vi "SLM_Calibrator.vi"() -> ()   [LabVIEW 2011]
uses:
  <vilib>/userDefined/High Color/IMAQdx.ctl
  <vilib>/vision/driver/NI_Vision_Acquisition_Software.lvlib
panel:
  in  "Xoffset2":dbl=4.136690647482014
  in  "Yoffset2":dbl=4.136690647482014
  in  "Yoffset1":dbl=6.374501992031872 caption="Fine:"
  in  "Xoffset1":dbl=6.374501992031872 caption="Fine:"
  in  "Direct to MatLab":bool
  out "ph_2_135":bool
  out "ph_2_45":bool
  out "ph_1_135":bool
  out "ph_1_45":bool
  out "I_2":bool
  out "I_1":bool
  out "0_255":dbl[](array[numeric])
  out "SupportFiles path":path
  out "I2":dbl[](array[numeric])
  out "ph2 135":dbl[](array[numeric])
  out "ph2 45":dbl[](array[numeric])
  out "I1":dbl[](array[numeric])
  out "ph1 135":dbl[](array[numeric])
  out "ph1_45":dbl[](array[numeric])
  in  "Ready?\nCalibrate!":bool caption="Stop (F)"
  in  "Active2":bool=TRUE caption="Hide/Show (Show)"
  in  "Active1":bool=TRUE caption="Hide/Show (Show)"
  in  "Yc1":dbl(slide)=2.231075697211155 scale=0.0..10.0
  in  "Yf1:":dbl(slide)=6.374501992031872 caption="Fine:" scale=0.0..10.0
  in  "Xc1":dbl(slide)=8.37920489296636 caption="X position" scale=0.0..10.0
  in  "Xf1:":dbl(slide)=9.026845637583893 caption="Fine:" scale=0.0..10.0
  out "Yi1":dbl caption="Y position"
  out "Xi1":dbl
  in  "Xc2":dbl(slide)=1.1180124223602483 caption="X position" scale=0.0..10.0
  in  "Xf2:":dbl(slide)=2.651006711409396 caption="Fine:" scale=0.0..10.0
  out "Xi2":dbl
  in  "Yf2:":dbl(slide)=5.467625899280575 caption="Fine:" scale=0.0..10.0
  in  "Yc2":dbl(slide)=4.136690647482014 scale=0.0..10.0
  out "Yi2":dbl caption="Y position"
  out "CGH_x\nSLM1":T1(plugin-control)
  out "CGH_y\nSLM2":T1(plugin-control)
  in  "Gradient1":bool
  in  "Gradient2":bool
  out "Status:":string
  in  "Label:":string
  out "Images done":dbl(slide) scale=0.0..256.0
  in  "Tab Control":T2(tab)
  out "CCD":T1(plugin-control)
  out "phase SLM1":cluster{dbl, dbl}[](graph)
  out "phase SLM2":cluster{dbl, dbl}[](graph)
  out "amplitude SLM2":cluster{dbl, dbl}[](graph)
  out "amplitude SLM1":cluster{dbl, dbl}[](graph)
  in  "Enough":bool caption="Stop (F)"
  out "smoother plot":cluster{dbl, dbl}[](graph)
  in  "Again":bool caption="Stop (F)"
  out "polar SLM1":picture
  out "polar SLM2":picture
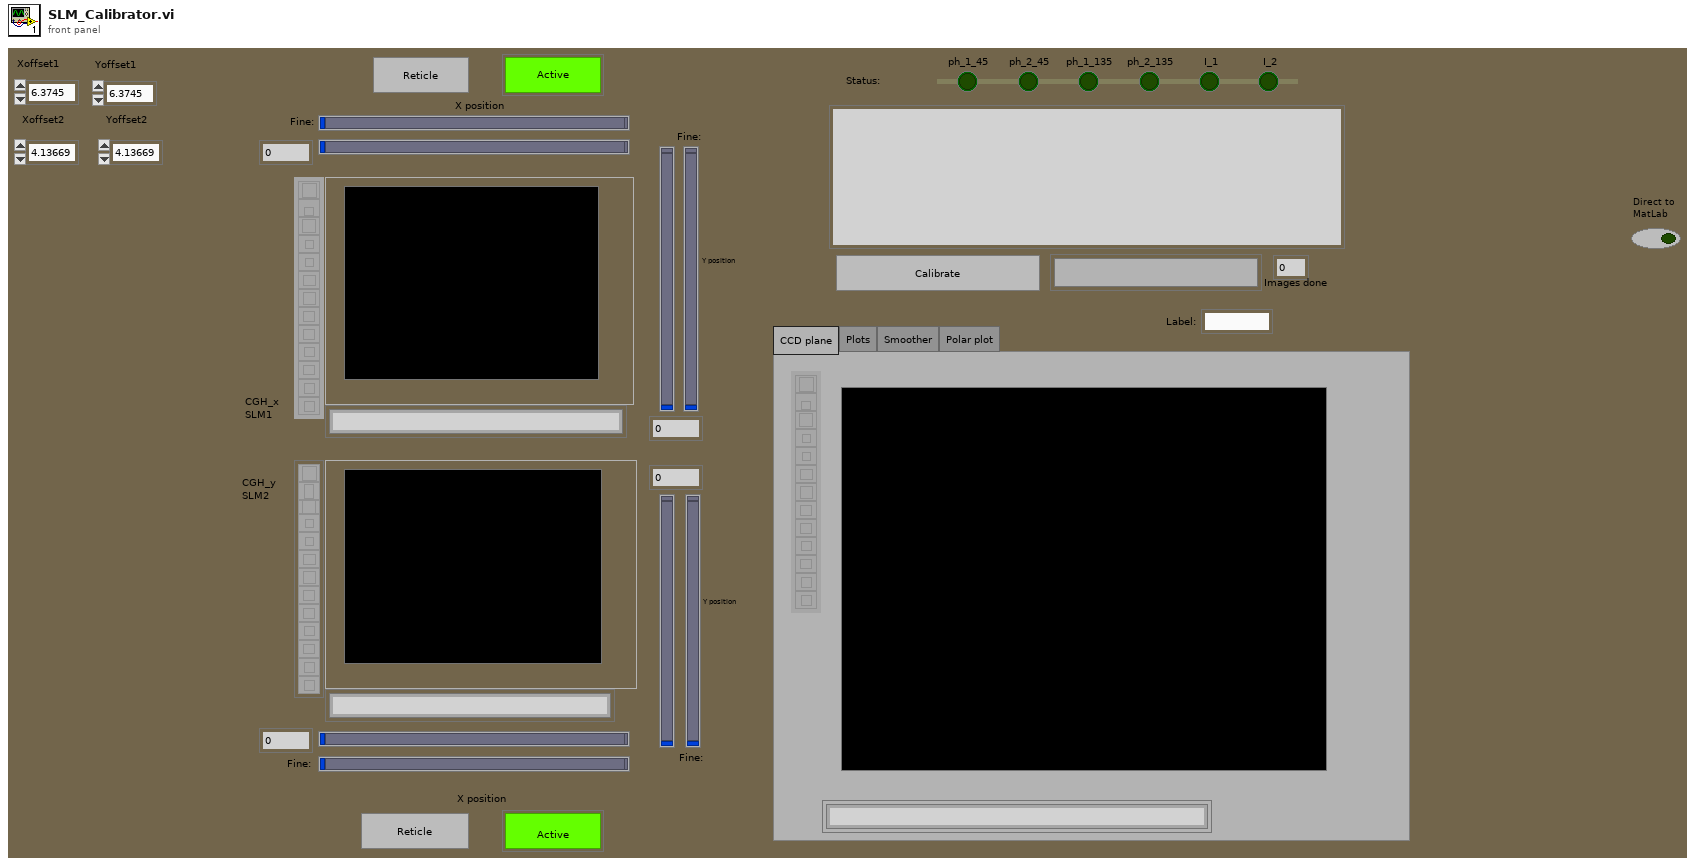
[diagram p1: front panel]
types:
  T1 = typedef "IMAQ Image.ctl" = refnum<image>
  T2 = enum32{"CCD plane", "Plots", "Smoother", "Polar plot"}
  T3 = typedef "IMAQdx.ctl" = refnum<k21>
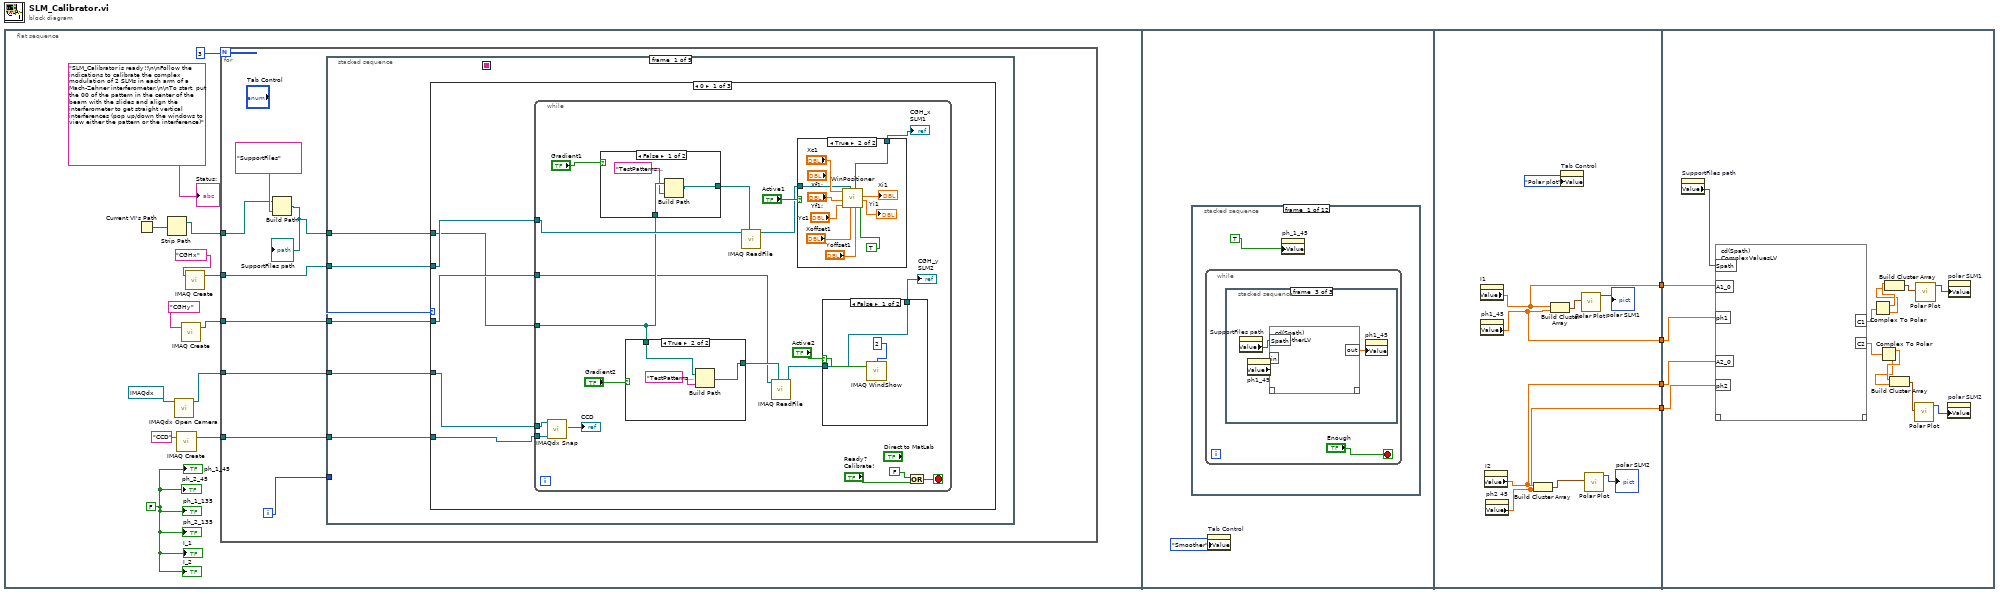
[diagram p0: block diagram]
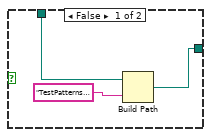
[diagram p2: hidden frame]
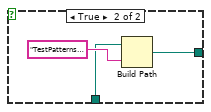
[diagram p3: hidden frame]
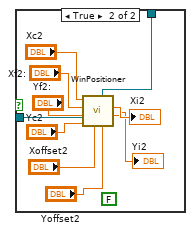
[diagram p4: hidden frame]
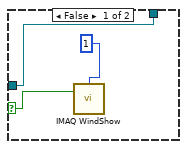
[diagram p5: hidden frame]
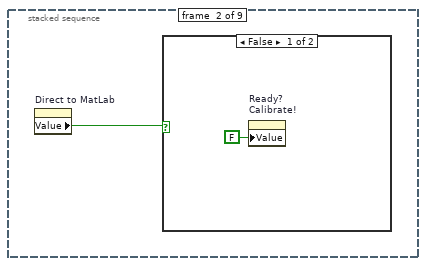
[diagram p8: hidden frame]
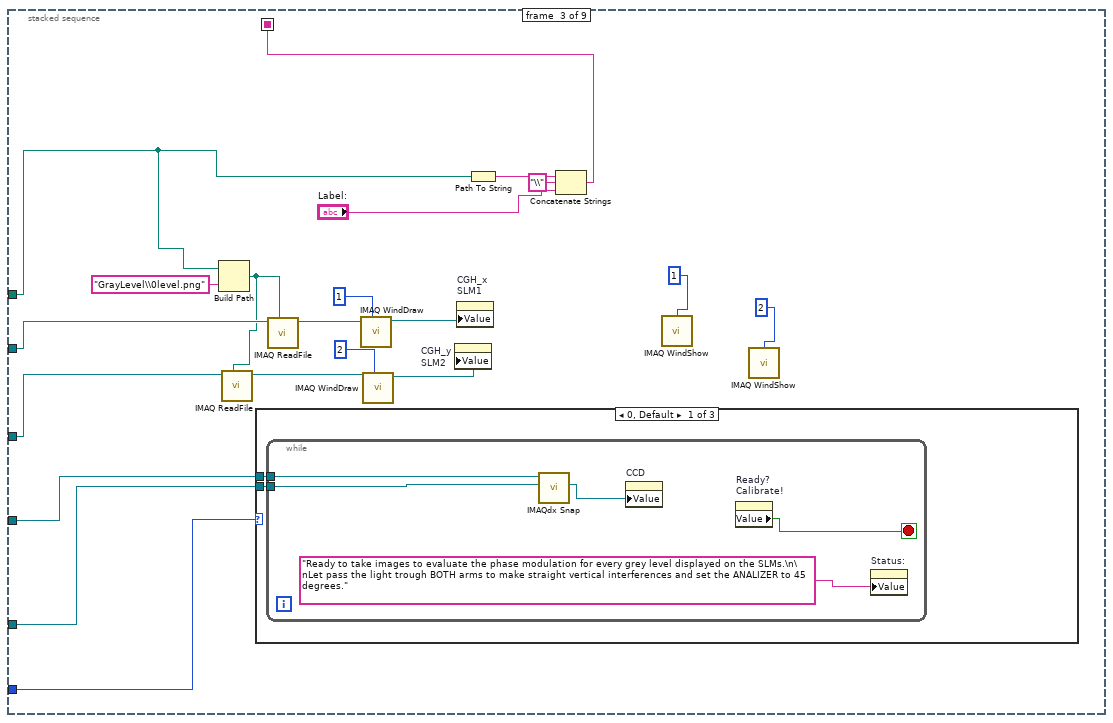
[diagram p10: hidden frame]
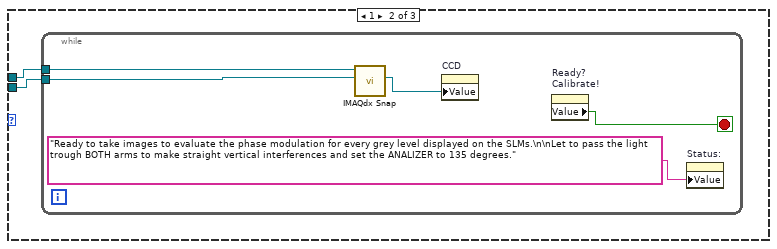
[diagram p11: hidden frame]
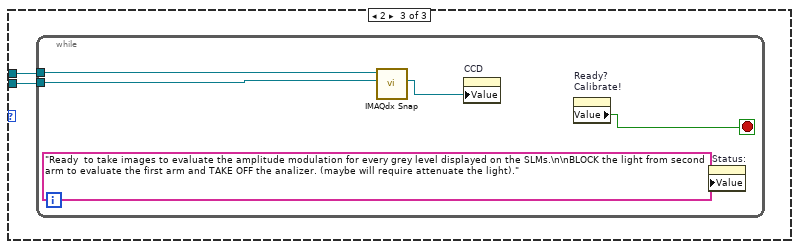
[diagram p12: hidden frame]
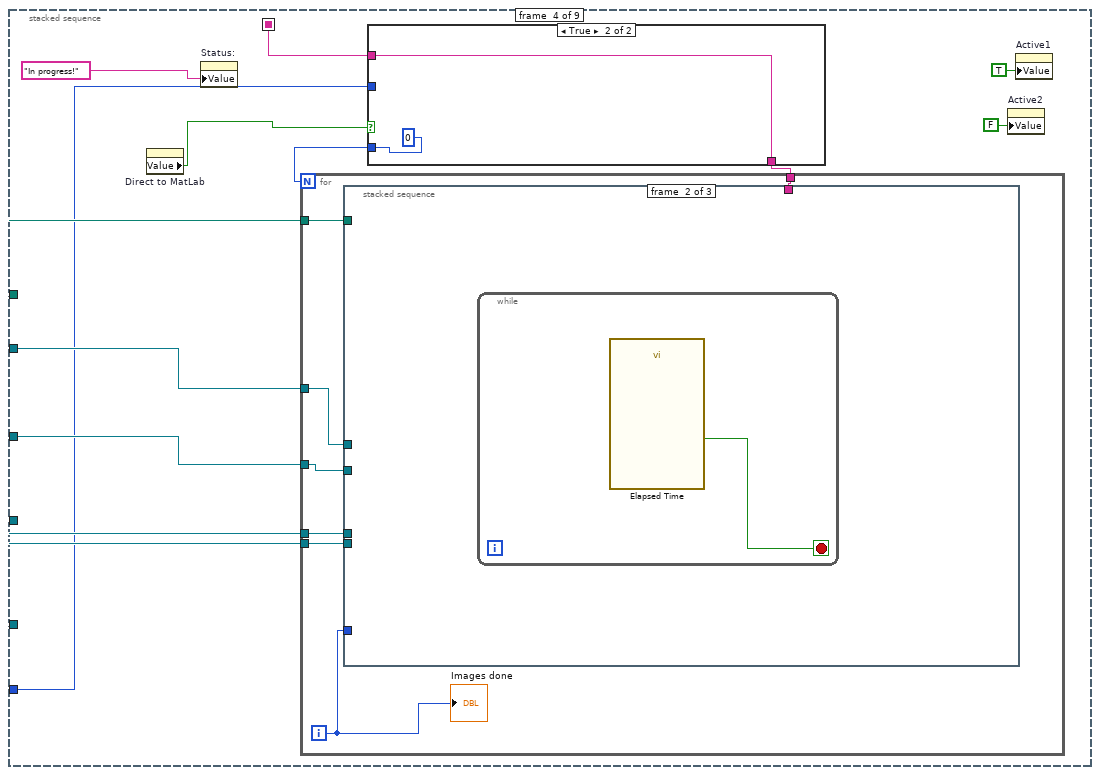
[diagram p13: hidden frame]
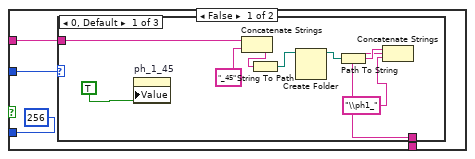
[diagram p14: hidden frame]
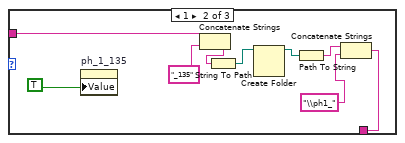
[diagram p15: hidden frame]
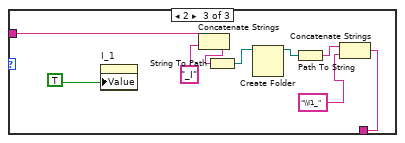
[diagram p16: hidden frame]
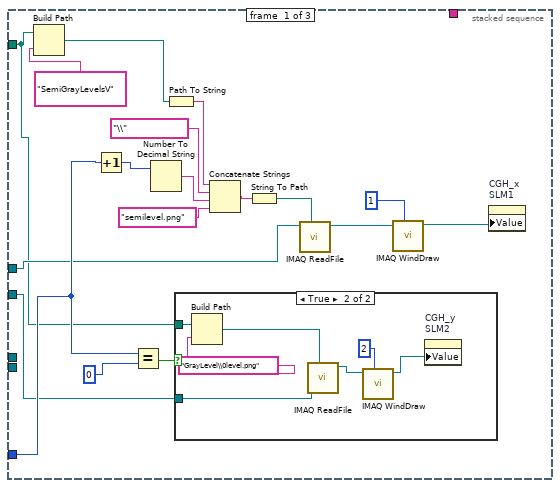
[diagram p17: hidden frame]
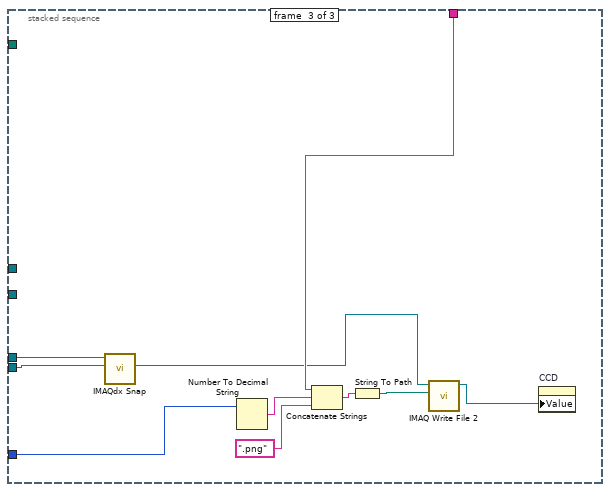
[diagram p19: hidden frame]
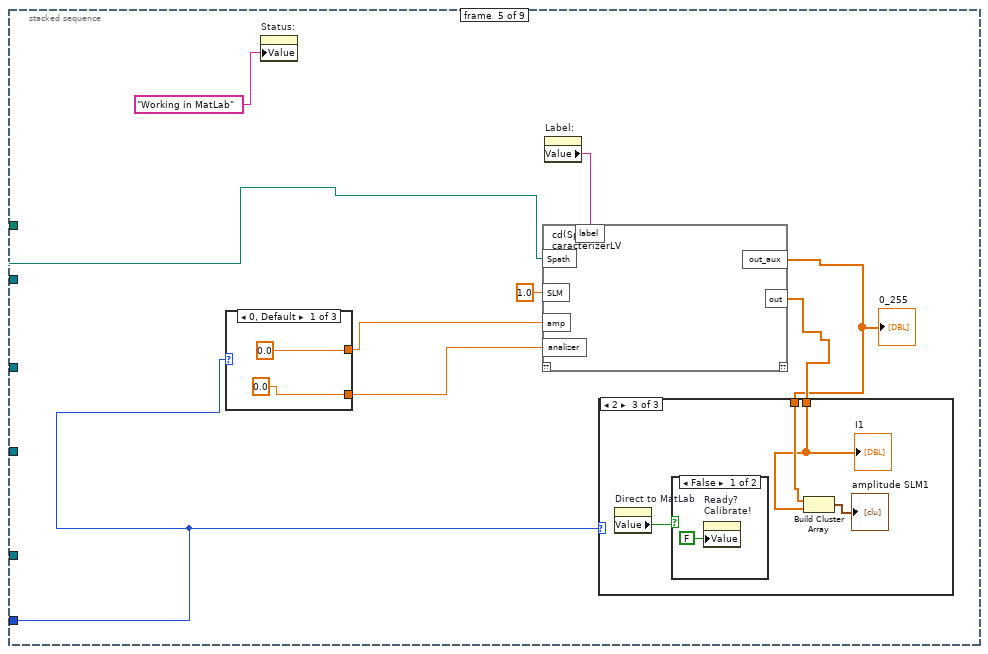
[diagram p20: hidden frame]
diagram:
  n1 = flat-sequence {
    tunnel: [w477] -> w4
    tunnel: [w476] -> w3
    tunnel: [w475] -> w2
    tunnel: [w474] -> w1
    tunnel: w4 -> [w493]
    tunnel: w3 -> [w492]
    tunnel: w2 -> [w495]
    tunnel: w1 -> [w494]
    frame #0 {
      w5 = FALSE ("x")
      n2 = Current VI's Path() -> (path=w11:path)
      n3 = Strip Path(path=w11) -> (stripped path=w10:path)  [unwired: 1 out]
      n4 = call <vilib>:"IMAQdx Open Camera.vi"("Session In"=T3 "cam0") -> ("Session Out"=w6:T3)  [unwired: 9 in, 1 out]
      n5 = call "IMAQ Create"("Image Name"="CCD") -> ("New Image"=w7:T1)  [unwired: 4 in, 1 out]
      n6 = call "IMAQ Create"("Image Name"="CGHy") -> ("New Image"=w13:T1)  [unwired: 4 in, 1 out]
      n7 = call "IMAQ Create"("Image Name"="CGHx") -> ("New Image"=w14:T1)  [unwired: 4 in, 1 out]
      n8 = for {
        N: 3 -> [_]
        tunnel: w14 -> [w25]
        tunnel: w13 -> [w24]
        tunnel: w10 -> [w19]
        tunnel: w7 -> [w23]
        tunnel: w6 -> [w22]
        i -> [w21]
        n9 = Build Path(base path=w19, name or relative path="SupportFiles") -> (appended path=w18:path)
        "SupportFiles path" <- w18
        n10 = stacked-sequence {
          seq-local: [_ _ w111 _ _ _ _ _ _] -> [_ _ _ w146 _ _ w272 _ _]
          tunnel: w24 -> [w30 _ w97 w148 _ _ w277 _ _]
          tunnel: w25 -> [w31 _ w100 w149 _ _ w278 _ _]
          tunnel: w21 -> [w29 _ w115 w142 w226 w257 w273 w349 w372]
          tunnel: w18 -> [w28 _ w105 w145 w233 _ w279 w351 _]
          tunnel: w23 -> [w27 _ w110 w143 _ w256 w275 _ _]
          tunnel: w22 -> [w26 _ w96 w144 _ w255 w276 _ _]
          frame #0 {
            n11 = case shown="0" w29 {
              tunnel: w31 -> [w34 _ _]
              tunnel: w30 -> [w33 _ _]
              tunnel: w28 -> [w32 _ _]
              tunnel: w27 -> [w36 _ _]
              tunnel: w26 -> [w35 _ _]
              frame 0 {
                n12 = while {
                  tunnel: w35 -> [w55]
                  tunnel: w36 -> [w54]
                  tunnel: w34 -> [w47]
                  tunnel: w33 -> [w40]
                  tunnel: w32 -> [w43]
                  stop <- w52 stop-if-true
                  n13 = call <vilib>:"IMAQdx Snap.vi"("Image In"=w54, "Session In"=w55) -> ("Image Out"=→"CCD":T1)  [unwired: 7 in, 2 out]
                  n14 = case shown="False" "Gradient1" {
                    tunnel: w43 -> [w64 w66]
                    tunnel: [w62 w65] -> w44
                    frame False {
                      n15 = Build Path(base path=w64, name or relative path="TestPatterns\\test_pattern.bmp") -> (appended path=w62:path)
                    }
                    frame True {
                      n16 = Build Path(base path=w66, name or relative path="TestPatterns\\test_pattern2V.png") -> (appended path=w65:path)
                    }
                  }
                  n17 = case shown="True" "Gradient2" {
                    tunnel: [w57 w59] -> w41
                    tunnel: w43 -> [w56 w60]
                    frame False {
                      n18 = Build Path(base path=w56, name or relative path="TestPatterns\\test_pattern.bmp") -> (appended path=w57:path)
                    }
                    frame True {
                      n19 = Build Path(base path=w60, name or relative path="TestPatterns\\test_pattern2.png") -> (appended path=w59:path)
                    }
                  }
                  n20 = call "IMAQ ReadFile"("File Path"=w44, "Image"=w47) -> ("Image Out"=w38:T1)  [unwired: 5 in, 4 out]
                  n21 = call "IMAQ ReadFile"("File Path"=w41, "Image"=w40) -> ("Image Out"=w49:T1)  [unwired: 5 in, 4 out]
                  n22 = case shown="True" "Active1" {
                    selector: "Active1" -> [w83 _]
                    tunnel: w38 -> [w81 w85]
                    tunnel: [w81 w84] -> w37
                    frame False {
                      n23 = call "IMAQ WindShow"("Hide/Show (Show)"=w83, "Window Number (0...15)"=1) -> ()  [unwired: 4 in, 3 out]
                    }
                    frame True {
                      n24 = call "WinPositioner.vi"("Display?"=TRUE, "Yoffset 2"="Yoffset1", "Xoffset"="Xoffset1", "Image"=w85, "Y position"="Yc1", "Fine Y position"="Yf1:", "X position"="Xc1") -> ("Y position"=→"Yi1":dbl, "X position"=→"Xi1":dbl, "CGH_x"=w84:T1)  [unwired: 2 in]
                    }
                  }
                  "CGH_x\nSLM1" <- w37
                  n25 = case shown="False" "Active2" {
                    selector: "Active2" -> [w70 _]
                    tunnel: [w68 w71] -> w50
                    tunnel: w49 -> [w68 w72]
                    frame False {
                      n26 = call "IMAQ WindShow"("Hide/Show (Show)"=w70, "Window Number (0...15)"=2) -> ()  [unwired: 4 in, 3 out]
                    }
                    frame True {
                      (unwired) FALSE ("Display?")
                      n27 = call "WinPositioner.vi"("Yoffset 2"="Yoffset2", "Xoffset"="Xoffset2", "Image"=w72, "Y position"="Yc2", "Fine Y position"="Yf2:", "Fine X position"="Xf2:", "X position"="Xc2") -> ("Y position"=→"Yi2":dbl, "X position"=→"Xi2":dbl, "CGH_x"=w71:T1)  [unwired: 2 in]
                    }
                  }
                  "CGH_y\nSLM2" <- w50
                  n28 = Or(x=FALSE, y="Ready?\nCalibrate!") -> (x .or. y?=w52:bool)
                }
              }
              frame 2 {
              }
              frame 1, Default {
              }
            }
          }
          frame #1 {
            n29 = property on="Direct to MatLab" class="Bool (strict)"() -> ("Value"=w94:bool)  [unwired: 2 in, 2 out]
            n30 = case shown="False" w94 {
              frame False {
                n31 = property on="Ready?\nCalibrate!" class="Bool (strict)"("Value"=FALSE ("Ready?\nCalibrate!")) -> ()  [unwired: 2 in, 2 out]
              }
              frame True {
              }
            }
          }
          frame #2 {
            n32 = Build Path(base path=w105, name or relative path="GrayLevel\\0level.png") -> (appended path=w98:path)
            n33 = call "IMAQ ReadFile"("File Path"=w98, "Image"=w97) -> ("Image Out"=w99:T1)  [unwired: 5 in, 4 out]
            n34 = case shown="0, Default" w115 {
              tunnel: w96 -> [w117 w124 w131]
              tunnel: w110 -> [w116 w123 w130]
              frame 0, Default {
                n35 = while {
                  tunnel: w117 -> [w121]
                  tunnel: w116 -> [w120]
                  stop <- w118 stop-if-true
                  n36 = call <vilib>:"IMAQdx Snap.vi"("Image In"=w120, "Session In"=w121) -> ("Image Out"=w119:T1)  [unwired: 7 in, 2 out]
                  n37 = property on="CCD" class="ImageControl"("Value"=w119) -> ()  [unwired: 2 in, 2 out]
                  n38 = property on="Ready?\nCalibrate!" class="Bool (strict)"() -> ("Value"=w118:bool)  [unwired: 2 in, 2 out]
                  n39 = property on="Status:" class="Str"("Value"="Ready to take images to evaluate the phase modulation for every grey level displayed on the SLMs.\n\nLet pass the light trough BOTH arms to make straight vertical interferences and set the ANALIZER to 45 degrees." ("message")) -> ()  [unwired: 2 in, 2 out]
                }
              }
              frame 1 {
                n40 = while {
                  tunnel: w124 -> [w129]
                  tunnel: w123 -> [w128]
                  stop <- w126 stop-if-true
                  n41 = call <vilib>:"IMAQdx Snap.vi"("Image In"=w128, "Session In"=w129) -> ("Image Out"=w127:T1)  [unwired: 7 in, 2 out]
                  n42 = property on="CCD" class="ImageControl"("Value"=w127) -> ()  [unwired: 2 in, 2 out]
                  n43 = property on="Ready?\nCalibrate!" class="Bool (strict)"() -> ("Value"=w126:bool)  [unwired: 2 in, 2 out]
                  n44 = property on="Status:" class="Str"("Value"="Ready to take images to evaluate the phase modulation for every grey level displayed on the SLMs.\n\nLet to pass the light trough BOTH arms to make straight vertical interferences and set the ANALIZER to 135 degrees." ("message")) -> ()  [unwired: 2 in, 2 out]
                }
              }
              frame 2 {
                n45 = while {
                  tunnel: w131 -> [w135]
                  tunnel: w130 -> [w134]
                  stop <- w132 stop-if-true
                  n46 = call <vilib>:"IMAQdx Snap.vi"("Image In"=w134, "Session In"=w135) -> ("Image Out"=w133:T1)  [unwired: 7 in, 2 out]
                  n47 = property on="CCD" class="ImageControl"("Value"=w133) -> ()  [unwired: 2 in, 2 out]
                  n48 = property on="Ready?\nCalibrate!" class="Bool (strict)"() -> ("Value"=w132:bool)  [unwired: 2 in, 2 out]
                  n49 = property on="Status:" class="Str"("Value"="Ready  to take images to evaluate the amplitude modulation for every grey level displayed on the SLMs.\n\nBLOCK the light from second arm to evaluate the first arm and TAKE OFF the analizer. (maybe will require attenuate the light)." ("message")) -> ()  [unwired: 2 in, 2 out]
                }
              }
            }
            n50 = call "IMAQ ReadFile"("File Path"=w98, "Image"=w100) -> ("Image Out"=w101:T1)  [unwired: 5 in, 4 out]
            n51 = call "IMAQ WindDraw"("Window Number (0...15)"=1, "Image"=w101) -> ("Image Out (duplicate)"=w106:T1)  [unwired: 8 in, 1 out]
            n52 = call "IMAQ WindDraw"("Window Number (0...15)"=2, "Image"=w99) -> ("Image Out (duplicate)"=w102:T1)  [unwired: 8 in, 1 out]
            n53 = property on="CGH_y\nSLM2" class="ImageControl"("Value"=w102) -> ()  [unwired: 2 in, 2 out]
            n54 = property on="CGH_x\nSLM1" class="ImageControl"("Value"=w106) -> ()  [unwired: 2 in, 2 out]
            n55 = Path To String(path=w105) -> (string=w114:string)
            n56 = Concatenate Strings(w114, "\\" ("string"), "Label:") -> (w111:string)
            n57 = call "IMAQ WindShow"("Window Number (0...15)"=1) -> ()  [unwired: 5 in, 3 out]
            n58 = call "IMAQ WindShow"("Window Number (0...15)"=2) -> ()  [unwired: 5 in, 3 out]
          }
          frame #3 {
            n59 = property on="Direct to MatLab" class="Bool (strict)"() -> ("Value"=w138:bool)  [unwired: 2 in, 2 out]
            n60 = property on="Status:" class="Str"("Value"="In progress!" ("Status")) -> ()  [unwired: 2 in, 2 out]
            n61 = case shown="True" w138 {
              tunnel: [w153 w181] -> w147
              tunnel: w146 -> [w152 w181]
              tunnel: w142 -> [w151 _]
              tunnel: [256 0] -> w137
              frame False {
                n62 = case shown="0, Default" w151 {
                  tunnel: [w156 w165 w174] -> w153
                  tunnel: w152 -> [w155 w164 w173]
                  frame 0, Default {
                    n63 = property on="ph_1_45" class="Bool (strict)"("Value"=TRUE ("135º")) -> ()  [unwired: 2 in, 2 out]
                    n64 = Concatenate Strings(w155, "_45" ("string")) -> (w161:string)
                    n65 = String To Path(string=w161) -> (path=w160:path)
                    n66 = Create Folder(path (use dialog)=w160) -> (created path=w159:path)  [unwired: 2 in, 2 out]
                    n67 = Path To String(path=w159) -> (string=w158:string)
                    n68 = Concatenate Strings(w158, "\\ph1_") -> (w156:string)
                  }
                  frame 1 {
                    n69 = property on="ph_1_135" class="Bool (strict)"("Value"=TRUE ("135º")) -> ()  [unwired: 2 in, 2 out]
                    n70 = Concatenate Strings(w164, "_135" ("string")) -> (w170:string)
                    n71 = String To Path(string=w170) -> (path=w169:path)
                    n72 = Create Folder(path (use dialog)=w169) -> (created path=w168:path)  [unwired: 2 in, 2 out]
                    n73 = Path To String(path=w168) -> (string=w167:string)
                    n74 = Concatenate Strings(w167, "\\ph1_") -> (w165:string)
                  }
                  frame 2 {
                    n75 = property on="I_1" class="Bool (strict)"("Value"=TRUE ("135º")) -> ()  [unwired: 2 in, 2 out]
                    n76 = Concatenate Strings(w173, "_I" ("string")) -> (w179:string)
                    n77 = String To Path(string=w179) -> (path=w178:path)
                    n78 = Create Folder(path (use dialog)=w178) -> (created path=w177:path)  [unwired: 2 in, 2 out]
                    n79 = Path To String(path=w177) -> (string=w176:string)
                    n80 = Concatenate Strings(w176, "\\I1_") -> (w174:string)
                  }
                }
              }
              frame True {
              }
            }
            n81 = for {
              N: w137 -> [_]
              tunnel: w149 -> [w189]
              tunnel: w148 -> [w188]
              tunnel: w147 -> [w186]
              tunnel: w145 -> [w185]
              tunnel: w144 -> [w184]
              tunnel: w143 -> [w183]
              i -> [w187]
              n82 = stacked-sequence {
                tunnel: w187 -> [w207 _ w221]
                tunnel: w189 -> [w206 _ _]
                tunnel: w188 -> [w191 _ _]
                tunnel: w186 -> [_ _ w220]
                tunnel: w185 -> [w192 _ _]
                tunnel: w184 -> [_ _ w218]
                tunnel: w183 -> [_ _ w217]
                frame #0 {
                  n83 = Build Path(base path=w192, name or relative path="SemiGrayLevelsV") -> (appended path=w193:path)
                  n84 = Increment(x=w207) -> (x+1=w200:i32)
                  n85 = Equal?(x=w207, y=0) -> (x = y?=w196:bool)
                  n86 = Number To Decimal String(number=w200) -> (decimal integer string=w201:string)  [unwired: 1 in]
                  n87 = Path To String(path=w193) -> (string=w202:string)
                  n88 = case shown="True" w196 {
                    tunnel: w191 -> [_ w212]
                    tunnel: w192 -> [_ w211]
                    frame False {
                    }
                    frame True {
                      n89 = Build Path(base path=w211, name or relative path="GrayLevel\\0level.png") -> (appended path=w209:path)
                      n90 = call "IMAQ ReadFile"("File Path"=w209, "Image"=w212) -> ("Image Out"=w214:T1)  [unwired: 5 in, 4 out]
                      n91 = call "IMAQ WindDraw"("Window Number (0...15)"=2, "Image"=w214) -> ("Image Out (duplicate)"=w208:T1)  [unwired: 8 in, 1 out]
                      n92 = property on="CGH_y\nSLM2" class="ImageControl"("Value"=w208) -> ()  [unwired: 2 in, 2 out]
                    }
                  }
                  n93 = Concatenate Strings(w202, "\\", w201, "semilevel.png") -> (w198:string)
                  n94 = String To Path(string=w198) -> (path=w197:path)
                  n95 = call "IMAQ ReadFile"("File Path"=w197, "Image"=w206) -> ("Image Out"=w205:T1)  [unwired: 5 in, 4 out]
                  n96 = call "IMAQ WindDraw"("Window Number (0...15)"=1, "Image"=w205) -> ("Image Out (duplicate)"=w190:T1)  [unwired: 8 in, 1 out]
                  n97 = property on="CGH_x\nSLM1" class="ImageControl"("Value"=w190) -> ()  [unwired: 2 in, 2 out]
                }
                frame #1 {
                  n98 = while {
                    stop <- w215 stop-if-true
                    n99 = call "Elapsed Time"() -> ("Time has Elapsed"=w215:bool)  [unwired: 12 in, 7 out]
                  }
                }
                frame #2 {
                  n100 = call <vilib>:"IMAQdx Snap.vi"("Image In"=w217, "Session In"=w218) -> ("Image Out"=w219:T1)  [unwired: 7 in, 2 out]
                  n101 = Number To Decimal String(number=w221) -> (decimal integer string=w223:string)  [unwired: 1 in]
                  n102 = Concatenate Strings(w220, w223, ".png") -> (w225:string)
                  n103 = String To Path(string=w225) -> (path=w222:path)
                  n104 = call-poly "IMAQ Write File 2"("File Path"=w222, "Image"=w219) -> ("Image Out (duplicate)"=w216:T1)  [unwired: 8 in, 1 out]
                  n105 = property on="CCD" class="ImageControl"("Value"=w216) -> ()  [unwired: 2 in, 2 out]
                }
              }
              "Images done" <- w187
            }
            n106 = property on="Active2" class="Bool (strict)"("Value"=FALSE ("Active2")) -> ()  [unwired: 2 in, 2 out]
            n107 = property on="Active1" class="Bool (strict)"("Value"=TRUE ("Active1")) -> ()  [unwired: 2 in, 2 out]
          }
          frame #4 {
            n108 = case shown="0, Default" w226 {
              tunnel: [0.0 ("Real") 0.0 ("Real") 1.0 ("Real")] -> w231
              tunnel: [0.0 ("Real") 1.0 ("Real") 0.0 ("Real")] -> w230
              frame 0, Default {
              }
              frame 1 {
              }
              frame 2 {
              }
            }
            n109 = property on="Status:" class="Str"("Value"="Working in MatLab" ("Status")) -> ()  [unwired: 2 in, 2 out]
            n110 = property on="Label:" class="Str"() -> ("Value"=w232:string)  [unwired: 2 in, 2 out]
            n111 = script code="cd(Spath)\ncaracterizerLV"("SLM"=1.0 ("Real"), "amp"=w231, "Spath"=w233, "analizer"=w230, "label"=w232) -> ("out"=w229:dbl[], "out_aux"=w228:dbl[])  [unwired: 1 in, 1 out]
            "0_255" <- w228
            n112 = case shown="2" w226 {
              tunnel: w228 -> [w242 w245 w250]
              tunnel: w229 -> [w241 w246 w249]
              frame 0, Default {
                n113 = Build Cluster Array(w242, w241) -> (→"phase SLM1":cluster{dbl, dbl}[])
                "ph1_45" <- w241
              }
              frame 1 {
                n114 = Build Cluster Array(w245, w246) -> (w244:cluster{dbl, dbl}[])
                n115 = property on="phase SLM1" class="XYGraph (strict)"("Value"=w244) -> ()  [unwired: 2 in, 2 out]
                "ph1 135" <- w246
              }
              frame 2 {
                n116 = property on="Direct to MatLab" class="Bool (strict)"() -> ("Value"=w247:bool)  [unwired: 2 in, 2 out]
                n117 = case shown="False" w247 {
                  frame False {
                    n118 = property on="Ready?\nCalibrate!" class="Bool (strict)"("Value"=FALSE ("Ready?\nCalibrate!")) -> ()  [unwired: 2 in, 2 out]
                  }
                  frame True {
                  }
                }
                n119 = Build Cluster Array(w250, w249) -> (→"amplitude SLM1":cluster{dbl, dbl}[])
                "I1" <- w249
              }
            }
          }
          frame #5 {
            n120 = case shown="2" w257 {
              tunnel: w256 -> [_ _ w262]
              tunnel: w255 -> [_ _ w261]
              frame 0, Default {
                n121 = property on="Ready?\nCalibrate!" class="Bool (strict)"("Value"=TRUE ("Ready?\nCalibrate!")) -> ()  [unwired: 2 in, 2 out]
              }
              frame 1 {
                n122 = property on="Ready?\nCalibrate!" class="Bool (strict)"("Value"=TRUE ("Ready?\nCalibrate!")) -> ()  [unwired: 2 in, 2 out]
              }
              frame 2 {
                n123 = while {
                  tunnel: w262 -> [w265]
                  tunnel: w261 -> [w264]
                  stop <- w266 stop-if-true
                  n124 = call <vilib>:"IMAQdx Snap.vi"("Image In"=w265, "Session In"=w264) -> ("Image Out"=w263:T1)  [unwired: 7 in, 2 out]
                  n125 = property on="CCD" class="ImageControl"("Value"=w263) -> ()  [unwired: 2 in, 2 out]
                  n126 = property on="Ready?\nCalibrate!" class="Bool (strict)"() -> ("Value"=w266:bool)  [unwired: 2 in, 2 out]
                  n127 = property on="Status:" class="Str"("Value"="Ready  to take images to evaluate the amplitude modulation for every grey level displayed on the SLMs.\n\nBLOCK the light from second arm to evaluate the first arm and TAKE OFF the analizer. (maybe will require attenuate the light)." ("message")) -> ()  [unwired: 2 in, 2 out]
                }
              }
            }
            n128 = property on="Tab Control" class="TabCtl (strict)"("Value"=T2."Plots" ("Tab Control")) -> ()  [unwired: 2 in, 2 out]
            n129 = property on="Images done" class="Slide (strict)"("Value"=0.0 ("Images done")) -> ()  [unwired: 2 in, 2 out]
            n130 = call "IMAQ WindShow"("Window Number (0...15)"=1) -> ()  [unwired: 5 in, 3 out]
            n131 = call "IMAQ WindShow"("Window Number (0...15)"=2) -> ()  [unwired: 5 in, 3 out]
          }
          frame #6 {
            n132 = property on="Direct to MatLab" class="Bool (strict)"() -> ("Value"=w268:bool)  [unwired: 2 in, 2 out]
            n133 = case shown="False" w268 {
              tunnel: [256 0] -> w280
              frame False {
              }
              frame True {
              }
            }
            n134 = property on="Status:" class="Str"("Value"="In progress!" ("Status")) -> ()  [unwired: 2 in, 2 out]
            n135 = case shown="1" w273 {
              tunnel: [w286 w292 w298] -> w274
              tunnel: w272 -> [w285 w291 w297]
              frame 0, Default {
                n136 = property on="ph_2_45" class="Bool (strict)"("Value"=TRUE ("135º")) -> ()  [unwired: 2 in, 2 out]
                n137 = Concatenate Strings(w285, "_45" ("string")) -> (w283:string)
                n138 = Concatenate Strings(w283, "\\ph2_") -> (w286:string)
              }
              frame 1 {
                n139 = property on="ph_2_135" class="Bool (strict)"("Value"=TRUE ("135º")) -> ()  [unwired: 2 in, 2 out]
                n140 = Concatenate Strings(w291, "_135" ("string")) -> (w289:string)
                n141 = Concatenate Strings(w289, "\\ph2_") -> (w292:string)
              }
              frame 2 {
                n142 = property on="I_2" class="Bool (strict)"("Value"=TRUE ("135º")) -> ()  [unwired: 2 in, 2 out]
                n143 = Concatenate Strings(w297, "_I" ("string")) -> (w295:string)
                n144 = Concatenate Strings(w295, "\\I2_") -> (w298:string)
              }
            }
            n145 = for {
              N: w280 -> [_]
              tunnel: w278 -> [w307]
              tunnel: w277 -> [w306]
              tunnel: w279 -> [w305]
              tunnel: w276 -> [w304]
              tunnel: w275 -> [w303]
              tunnel: w274 -> [w302]
              i -> [w301]
              n146 = stacked-sequence {
                tunnel: w301 -> [w325 _ w339]
                tunnel: w307 -> [w323 _ _]
                tunnel: w306 -> [w324 _ _]
                tunnel: w305 -> [w309 _ _]
                tunnel: w304 -> [_ _ w338]
                tunnel: w303 -> [_ _ w337]
                tunnel: w302 -> [_ _ w335]
                frame #0 {
                  n147 = Build Path(base path=w309, name or relative path="SemiGrayLevels") -> (appended path=w310:path)
                  n148 = Equal?(x=w325, y=0) -> (x = y?=w313:bool)
                  n149 = case shown="True" w313 {
                    tunnel: w324 -> [_ w331]
                    tunnel: w309 -> [_ w329]
                    frame False {
                    }
                    frame True {
                      n150 = Build Path(base path=w329, name or relative path="GrayLevel\\0level.png") -> (appended path=w327:path)
                      n151 = call "IMAQ ReadFile"("File Path"=w327, "Image"=w331) -> ("Image Out"=w332:T1)  [unwired: 5 in, 4 out]
                      n152 = call "IMAQ WindDraw"("Window Number (0...15)"=1, "Image"=w332) -> ("Image Out (duplicate)"=w326:T1)  [unwired: 8 in, 1 out]
                      n153 = property on="CGH_x\nSLM1" class="ImageControl"("Value"=w326) -> ()  [unwired: 2 in, 2 out]
                    }
                  }
                  n154 = Increment(x=w325) -> (x+1=w318:i32)
                  n155 = Number To Decimal String(number=w318) -> (decimal integer string=w319:string)  [unwired: 1 in]
                  n156 = Path To String(path=w310) -> (string=w320:string)
                  n157 = Concatenate Strings(w320, "\\", w319, "semilevel.png") -> (w316:string)
                  n158 = String To Path(string=w316) -> (path=w315:path)
                  n159 = call "IMAQ ReadFile"("File Path"=w315, "Image"=w323) -> ("Image Out"=w322:T1)  [unwired: 5 in, 4 out]
                  n160 = call "IMAQ WindDraw"("Window Number (0...15)"=2, "Image"=w322) -> ("Image Out (duplicate)"=w308:T1)  [unwired: 8 in, 1 out]
                  n161 = property on="CGH_y\nSLM2" class="ImageControl"("Value"=w308) -> ()  [unwired: 2 in, 2 out]
                }
                frame #1 {
                  n162 = while {
                    stop <- w333 stop-if-true
                    n163 = call "Elapsed Time2"() -> ("Time has Elapsed"=w333:bool)  [unwired: 12 in, 7 out]
                  }
                }
                frame #2 {
                  n164 = Number To Decimal String(number=w339) -> (decimal integer string=w341:string)  [unwired: 1 in]
                  n165 = Concatenate Strings(w335, w341, ".png") -> (w343:string)
                  n166 = String To Path(string=w343) -> (path=w340:path)
                  n167 = call <vilib>:"IMAQdx Snap.vi"("Image In"=w337, "Session In"=w338) -> ("Image Out"=w336:T1)  [unwired: 7 in, 2 out]
                  n168 = call-poly "IMAQ Write File 2"("File Path"=w340, "Image"=w336) -> ("Image Out (duplicate)"=w334:T1)  [unwired: 8 in, 1 out]
                  n169 = property on="CCD" class="ImageControl"("Value"=w334) -> ()  [unwired: 2 in, 2 out]
                }
              }
              n170 = property on="Images done" class="Slide (strict)"("Value"=w301) -> ()  [unwired: 2 in, 2 out]
            }
            n171 = property on="Active1" class="Bool (strict)"("Value"=FALSE ("Active2")) -> ()  [unwired: 2 in, 2 out]
            n172 = property on="Active2" class="Bool (strict)"("Value"=TRUE ("Active1")) -> ()  [unwired: 2 in, 2 out]
          }
          frame #7 {
            n173 = case shown="0, Default" w349 {
              tunnel: [0.0 ("Real") 0.0 ("Real") 1.0 ("Real")] -> w348
              tunnel: [0.0 ("Real") 1.0 ("Real") 0.0 ("Real")] -> w347
              frame 0, Default {
              }
              frame 1 {
              }
              frame 2 {
              }
            }
            n174 = property on="Status:" class="Str"("Value"="Working in MatLab" ("Status")) -> ()  [unwired: 2 in, 2 out]
            n175 = property on="Label:" class="Str"() -> ("Value"=w350:string)  [unwired: 2 in, 2 out]
            n176 = script code="cd(Spath)\ncaracterizerLV"("SLM"=0.0 ("Real"), "amp"=w348, "Spath"=w351, "analizer"=w347, "label"=w350) -> ("out"=w345:dbl[], "out_aux"=w346:dbl[])  [unwired: 1 in, 1 out]
            n177 = case shown="0, Default" w349 {
              tunnel: w345 -> [w359 w362 w367]
              tunnel: w346 -> [w360 w363 w366]
              frame 0, Default {
                n178 = Build Cluster Array(w360, w359) -> (→"phase SLM2":cluster{dbl, dbl}[])
                "ph2 45" <- w359
              }
              frame 1 {
                n179 = Build Cluster Array(w363, w362) -> (w364:cluster{dbl, dbl}[])
                n180 = property on="phase SLM2" class="XYGraph (strict)"("Value"=w364) -> ()  [unwired: 2 in, 2 out]
                "ph2 135" <- w362
              }
              frame 2 {
                n181 = Build Cluster Array(w366, w367) -> (→"amplitude SLM2":cluster{dbl, dbl}[])
                "I2" <- w367
              }
            }
          }
          frame #8 {
            n182 = Equal?(x=w372, y=2) -> (x = y?=w370:bool)
            n183 = case shown="True" w370 {
              frame False {
              }
              frame True {
                w376 = TRUE ("Close All Windows (False)")
                n184 = call "IMAQ WindClose"("Close All Windows (False)"=w376) -> ()  [unwired: 5 in, 1 out]
                n185 = property on="Status:" class="Str"("Value"="Working in MatLab to sum up the calibration.") -> ()  [unwired: 2 in, 2 out]
                n186 = call "IMAQ Dispose"("All Images? (No)"=w376) -> ()  [unwired: 5 in, 1 out]
              }
            }
            n187 = property on="Tab Control" class="TabCtl (strict)"("Value"=T2."Plots" ("Tab Control")) -> ()  [unwired: 2 in, 2 out]
            n188 = property on="Direct to MatLab" class="Bool (strict)"() -> ("Value"=w368:bool)  [unwired: 2 in, 2 out]
            n189 = case shown="False" w368 {
              frame False {
                n190 = property on="Ready?\nCalibrate!" class="Bool (strict)"("Value"=FALSE ("Ready?\nCalibrate!")) -> ()  [unwired: 2 in, 2 out]
              }
              frame True {
              }
            }
            n191 = property on="Images done" class="Slide (strict)"("Value"=0.0 ("Images done")) -> ()  [unwired: 2 in, 2 out]
          }
        }
      }
      "Status:" <- "SLM_Calibrator is ready!!\n\nFollow the indications to calibrate the complex modulation of 2 SLMs in each arm of a Mach-Zehner interferometer.\n\nTo start, put the 00 of the pattern in the center of the beam with the slides and align the interferometer to get straight vertical interferences (pop up/down the windows to view either the pattern or the interference)" ("String")
      "I_1" <- w5
      "ph_1_45" <- w5
      "ph_1_135" <- w5
      "I_2" <- w5
      "ph_2_45" <- w5
      "ph_2_135" <- w5
    }
    frame #1 {
      n192 = stacked-sequence {
        frame #0 {
          n193 = while {
            stop <- "Enough" stop-if-true
            n194 = stacked-sequence {
              frame #0 {
                n195 = while {
                  stop <- w382 stop-if-true
                  n196 = property on="0_255" class="Arr (strict)"() -> ("Value"=w385:dbl[])  [unwired: 2 in, 2 out]
                  n197 = property on="ph1_45" class="Arr (strict)"() -> ("Value"=w384:dbl[])  [unwired: 2 in, 2 out]
                  n198 = Build Cluster Array(w385, w384) -> (→"smoother plot":cluster{dbl, dbl}[])
                  n199 = property on="Enough" class="Bool (strict)"() -> ("Value"=w381:bool)  [unwired: 2 in, 2 out]
                  n200 = Or(x=w381, y="Again") -> (x .or. y?=w382:bool)
                }
              }
              frame #1 {
                n201 = property on="Again" class="Bool (strict)"("Value"=FALSE ("Again")) -> ()  [unwired: 2 in, 2 out]
              }
              frame #2 {
                n202 = property on="SupportFiles path" class="Path"() -> ("Value"=w389:path)  [unwired: 2 in, 2 out]
                n203 = property on="ph1_45" class="Arr (strict)"() -> ("Value"=w388:dbl[])  [unwired: 2 in, 2 out]
                n204 = script code="cd(Spath)\nsmootherLV"("Spath"=w389, "in"=w388) -> ("out"=w387:dbl[])  [unwired: 1 in, 1 out]
                n205 = property on="ph1_45" class="Arr (strict)"("Value"=w387) -> ()  [unwired: 2 in, 2 out]
              }
            }
          }
          n206 = property on="ph_1_45" class="Bool (strict)"("Value"=TRUE ("I1")) -> ()  [unwired: 2 in, 2 out]
        }
        frame #1 {
          w390 = FALSE ("Again")
          n207 = property on="ph_1_45" class="Bool (strict)"("Value"=w390) -> ()  [unwired: 2 in, 2 out]
          n208 = property on="Enough" class="Bool (strict)"("Value"=w390) -> ()  [unwired: 2 in, 2 out]
        }
        frame #2 {
          n209 = while {
            stop <- w392 stop-if-true
            n210 = stacked-sequence {
              frame #0 {
                n211 = while {
                  stop <- w396 stop-if-true
                  n212 = property on="0_255" class="Arr (strict)"() -> ("Value"=w398:dbl[])  [unwired: 2 in, 2 out]
                  n213 = property on="ph2 45" class="Arr (strict)"() -> ("Value"=w397:dbl[])  [unwired: 2 in, 2 out]
                  n214 = property on="Again" class="Bool (strict)"() -> ("Value"=w394:bool)  [unwired: 2 in, 2 out]
                  n215 = Build Cluster Array(w398, w397) -> (w395:cluster{dbl, dbl}[])
                  n216 = property on="Enough" class="Bool (strict)"() -> ("Value"=w393:bool)  [unwired: 2 in, 2 out]
                  n217 = property on="smoother plot" class="XYGraph (strict)"("Value"=w395) -> ()  [unwired: 2 in, 2 out]
                  n218 = Or(x=w393, y=w394) -> (x .or. y?=w396:bool)
                }
              }
              frame #1 {
                n219 = property on="Again" class="Bool (strict)"("Value"=FALSE ("Again")) -> ()  [unwired: 2 in, 2 out]
              }
              frame #2 {
                n220 = property on="SupportFiles path" class="Path"() -> ("Value"=w402:path)  [unwired: 2 in, 2 out]
                n221 = property on="ph2 45" class="Arr (strict)"() -> ("Value"=w401:dbl[])  [unwired: 2 in, 2 out]
                n222 = script code="cd(Spath)\nsmootherLV"("Spath"=w402, "in"=w401) -> ("out"=w400:dbl[])  [unwired: 1 in, 1 out]
                n223 = property on="ph2 45" class="Arr (strict)"("Value"=w400) -> ()  [unwired: 2 in, 2 out]
              }
            }
            n224 = property on="Enough" class="Bool (strict)"() -> ("Value"=w392:bool)  [unwired: 2 in, 2 out]
          }
          n225 = property on="ph_2_45" class="Bool (strict)"("Value"=TRUE ("ph1_45")) -> ()  [unwired: 2 in, 2 out]
        }
        frame #3 {
          w403 = FALSE ("Again")
          n226 = property on="Enough" class="Bool (strict)"("Value"=w403) -> ()  [unwired: 2 in, 2 out]
          n227 = property on="ph_2_45" class="Bool (strict)"("Value"=w403) -> ()  [unwired: 2 in, 2 out]
        }
        frame #4 {
          n228 = while {
            stop <- w405 stop-if-true
            n229 = stacked-sequence {
              frame #0 {
                n230 = while {
                  stop <- w409 stop-if-true
                  n231 = property on="ph1 135" class="Arr (strict)"() -> ("Value"=w410:dbl[])  [unwired: 2 in, 2 out]
                  n232 = property on="0_255" class="Arr (strict)"() -> ("Value"=w411:dbl[])  [unwired: 2 in, 2 out]
                  n233 = property on="Again" class="Bool (strict)"() -> ("Value"=w407:bool)  [unwired: 2 in, 2 out]
                  n234 = Build Cluster Array(w411, w410) -> (w408:cluster{dbl, dbl}[])
                  n235 = property on="Enough" class="Bool (strict)"() -> ("Value"=w406:bool)  [unwired: 2 in, 2 out]
                  n236 = property on="smoother plot" class="XYGraph (strict)"("Value"=w408) -> ()  [unwired: 2 in, 2 out]
                  n237 = Or(x=w406, y=w407) -> (x .or. y?=w409:bool)
                }
              }
              frame #1 {
                n238 = property on="Again" class="Bool (strict)"("Value"=FALSE ("Again")) -> ()  [unwired: 2 in, 2 out]
              }
              frame #2 {
                n239 = property on="SupportFiles path" class="Path"() -> ("Value"=w415:path)  [unwired: 2 in, 2 out]
                n240 = property on="ph1 135" class="Arr (strict)"() -> ("Value"=w414:dbl[])  [unwired: 2 in, 2 out]
                n241 = script code="cd(Spath)\nsmootherLV"("Spath"=w415, "in"=w414) -> ("out"=w413:dbl[])  [unwired: 1 in, 1 out]
                n242 = property on="ph1 135" class="Arr (strict)"("Value"=w413) -> ()  [unwired: 2 in, 2 out]
              }
            }
            n243 = property on="Enough" class="Bool (strict)"() -> ("Value"=w405:bool)  [unwired: 2 in, 2 out]
          }
          n244 = property on="ph_1_135" class="Bool (strict)"("Value"=TRUE ("ph1_135")) -> ()  [unwired: 2 in, 2 out]
        }
        frame #5 {
          w416 = FALSE ("Again")
          n245 = property on="ph_1_135" class="Bool (strict)"("Value"=w416) -> ()  [unwired: 2 in, 2 out]
          n246 = property on="Enough" class="Bool (strict)"("Value"=w416) -> ()  [unwired: 2 in, 2 out]
        }
        frame #6 {
          n247 = while {
            stop <- w418 stop-if-true
            n248 = stacked-sequence {
              frame #0 {
                n249 = while {
                  stop <- w422 stop-if-true
                  n250 = property on="0_255" class="Arr (strict)"() -> ("Value"=w424:dbl[])  [unwired: 2 in, 2 out]
                  n251 = property on="ph2 135" class="Arr (strict)"() -> ("Value"=w423:dbl[])  [unwired: 2 in, 2 out]
                  n252 = property on="Enough" class="Bool (strict)"() -> ("Value"=w420:bool)  [unwired: 2 in, 2 out]
                  n253 = Build Cluster Array(w424, w423) -> (w421:cluster{dbl, dbl}[])
                  n254 = property on="Again" class="Bool (strict)"() -> ("Value"=w419:bool)  [unwired: 2 in, 2 out]
                  n255 = property on="smoother plot" class="XYGraph (strict)"("Value"=w421) -> ()  [unwired: 2 in, 2 out]
                  n256 = Or(x=w419, y=w420) -> (x .or. y?=w422:bool)
                }
              }
              frame #1 {
                n257 = property on="Again" class="Bool (strict)"("Value"=FALSE ("Again")) -> ()  [unwired: 2 in, 2 out]
              }
              frame #2 {
                n258 = property on="SupportFiles path" class="Path"() -> ("Value"=w428:path)  [unwired: 2 in, 2 out]
                n259 = property on="ph2 135" class="Arr (strict)"() -> ("Value"=w427:dbl[])  [unwired: 2 in, 2 out]
                n260 = script code="cd(Spath)\nsmootherLV"("Spath"=w428, "in"=w427) -> ("out"=w426:dbl[])  [unwired: 1 in, 1 out]
                n261 = property on="ph2 135" class="Arr (strict)"("Value"=w426) -> ()  [unwired: 2 in, 2 out]
              }
            }
            n262 = property on="Enough" class="Bool (strict)"() -> ("Value"=w418:bool)  [unwired: 2 in, 2 out]
          }
          n263 = property on="ph_2_135" class="Bool (strict)"("Value"=TRUE ("I2")) -> ()  [unwired: 2 in, 2 out]
        }
        frame #7 {
          w429 = FALSE ("Again")
          n264 = property on="Enough" class="Bool (strict)"("Value"=w429) -> ()  [unwired: 2 in, 2 out]
          n265 = property on="ph_2_135" class="Bool (strict)"("Value"=w429) -> ()  [unwired: 2 in, 2 out]
        }
        frame #8 {
          n266 = while {
            stop <- w431 stop-if-true
            n267 = stacked-sequence {
              frame #0 {
                n268 = while {
                  stop <- w435 stop-if-true
                  n269 = property on="0_255" class="Arr (strict)"() -> ("Value"=w437:dbl[])  [unwired: 2 in, 2 out]
                  n270 = property on="I1" class="Arr (strict)"() -> ("Value"=w436:dbl[])  [unwired: 2 in, 2 out]
                  n271 = property on="Enough" class="Bool (strict)"() -> ("Value"=w433:bool)  [unwired: 2 in, 2 out]
                  n272 = Build Cluster Array(w437, w436) -> (w434:cluster{dbl, dbl}[])
                  n273 = property on="Again" class="Bool (strict)"() -> ("Value"=w432:bool)  [unwired: 2 in, 2 out]
                  n274 = property on="smoother plot" class="XYGraph (strict)"("Value"=w434) -> ()  [unwired: 2 in, 2 out]
                  n275 = Or(x=w432, y=w433) -> (x .or. y?=w435:bool)
                }
              }
              frame #1 {
                n276 = property on="Again" class="Bool (strict)"("Value"=FALSE ("Again")) -> ()  [unwired: 2 in, 2 out]
              }
              frame #2 {
                n277 = property on="SupportFiles path" class="Path"() -> ("Value"=w441:path)  [unwired: 2 in, 2 out]
                n278 = property on="I1" class="Arr (strict)"() -> ("Value"=w440:dbl[])  [unwired: 2 in, 2 out]
                n279 = script code="cd(Spath)\nsmootherLV"("Spath"=w441, "in"=w440) -> ("out"=w439:dbl[])  [unwired: 1 in, 1 out]
                n280 = property on="I1" class="Arr (strict)"("Value"=w439) -> ()  [unwired: 2 in, 2 out]
              }
            }
            n281 = property on="Enough" class="Bool (strict)"() -> ("Value"=w431:bool)  [unwired: 2 in, 2 out]
          }
          n282 = property on="I_1" class="Bool (strict)"("Value"=TRUE ("ph2_45")) -> ()  [unwired: 2 in, 2 out]
        }
        frame #9 {
          w442 = FALSE ("Again")
          n283 = property on="Enough" class="Bool (strict)"("Value"=w442) -> ()  [unwired: 2 in, 2 out]
          n284 = property on="I_1" class="Bool (strict)"("Value"=w442) -> ()  [unwired: 2 in, 2 out]
        }
        frame #10 {
          n285 = while {
            stop <- w444 stop-if-true
            n286 = stacked-sequence {
              frame #0 {
                n287 = while {
                  stop <- w448 stop-if-true
                  n288 = property on="0_255" class="Arr (strict)"() -> ("Value"=w450:dbl[])  [unwired: 2 in, 2 out]
                  n289 = property on="I2" class="Arr (strict)"() -> ("Value"=w449:dbl[])  [unwired: 2 in, 2 out]
                  n290 = property on="Enough" class="Bool (strict)"() -> ("Value"=w446:bool)  [unwired: 2 in, 2 out]
                  n291 = Build Cluster Array(w450, w449) -> (w447:cluster{dbl, dbl}[])
                  n292 = property on="Again" class="Bool (strict)"() -> ("Value"=w445:bool)  [unwired: 2 in, 2 out]
                  n293 = property on="smoother plot" class="XYGraph (strict)"("Value"=w447) -> ()  [unwired: 2 in, 2 out]
                  n294 = Or(x=w445, y=w446) -> (x .or. y?=w448:bool)
                }
              }
              frame #1 {
                n295 = property on="Again" class="Bool (strict)"("Value"=FALSE ("Again")) -> ()  [unwired: 2 in, 2 out]
              }
              frame #2 {
                n296 = property on="SupportFiles path" class="Path"() -> ("Value"=w454:path)  [unwired: 2 in, 2 out]
                n297 = property on="I2" class="Arr (strict)"() -> ("Value"=w453:dbl[])  [unwired: 2 in, 2 out]
                n298 = script code="cd(Spath)\nsmootherLV"("Spath"=w454, "in"=w453) -> ("out"=w452:dbl[])  [unwired: 1 in, 1 out]
                n299 = property on="I2" class="Arr (strict)"("Value"=w452) -> ()  [unwired: 2 in, 2 out]
              }
            }
            n300 = property on="Enough" class="Bool (strict)"() -> ("Value"=w444:bool)  [unwired: 2 in, 2 out]
          }
          n301 = property on="I_2" class="Bool (strict)"("Value"=TRUE ("ph2_135")) -> ()  [unwired: 2 in, 2 out]
        }
        frame #11 {
          w455 = FALSE ("Again")
          n302 = property on="ph2 135" class="Arr (strict)"() -> ("Value"=w469:dbl[])  [unwired: 2 in, 2 out]
          n303 = property on="ph2 45" class="Arr (strict)"() -> ("Value"=w470:dbl[])  [unwired: 2 in, 2 out]
          n304 = property on="ph1_45" class="Arr (strict)"() -> ("Value"=w471:dbl[])  [unwired: 2 in, 2 out]
          n305 = property on="I1" class="Arr (strict)"() -> ("Value"=w459:dbl[])  [unwired: 2 in, 2 out]
          n306 = property on="0_255" class="Arr (strict)"() -> ("Value"=w460:dbl[])  [unwired: 2 in, 2 out]
          n307 = property on="ph1 135" class="Arr (strict)"() -> ("Value"=w472:dbl[])  [unwired: 2 in, 2 out]
          n308 = property on="Enough" class="Bool (strict)"("Value"=w455) -> ()  [unwired: 2 in, 2 out]
          n309 = property on="I2" class="Arr (strict)"() -> ("Value"=w458:dbl[])  [unwired: 2 in, 2 out]
          n310 = Add(x=w470, y=w469) -> (x+y=w465:dbl[])
          n311 = property on="I_2" class="Bool (strict)"("Value"=w455) -> ()  [unwired: 2 in, 2 out]
          n312 = Add(x=w472, y=w471) -> (x+y=w468:dbl[])
          n313 = Multiply(x=w465, y=0.5) -> (x*y=w462:dbl[])
          n314 = Multiply(x=w468, y=0.5) -> (x*y=w463:dbl[])
          n315 = Build Cluster Array(w460, w463) -> (w464:cluster{dbl, dbl}[])
          n316 = Build Cluster Array(w460, w458) -> (w456:cluster{dbl, dbl}[])
          n317 = Build Cluster Array(w460, w459) -> (w457:cluster{dbl, dbl}[])
          n318 = Build Cluster Array(w460, w462) -> (w461:cluster{dbl, dbl}[])
          n319 = property on="ph1_45" class="Arr (strict)"("Value"=w463) -> ()  [unwired: 2 in, 2 out]
          n320 = property on="amplitude SLM2" class="XYGraph (strict)"("Value"=w456) -> ()  [unwired: 2 in, 2 out]
          n321 = property on="ph2 45" class="Arr (strict)"("Value"=w462) -> ()  [unwired: 2 in, 2 out]
          n322 = property on="amplitude SLM1" class="XYGraph (strict)"("Value"=w457) -> ()  [unwired: 2 in, 2 out]
          n323 = property on="phase SLM2" class="XYGraph (strict)"("Value"=w461) -> ()  [unwired: 2 in, 2 out]
          n324 = property on="phase SLM1" class="XYGraph (strict)"("Value"=w464) -> ()  [unwired: 2 in, 2 out]
        }
      }
      n325 = property on="Tab Control" class="TabCtl (strict)"("Value"=T2."Smoother" ("Tab Control")) -> ()  [unwired: 2 in, 2 out]
    }
    frame #2 {
      n326 = property on="I1" class="Arr (strict)"() -> ("Value"=w475:dbl[])  [unwired: 2 in, 2 out]
      n327 = property on="ph1_45" class="Arr (strict)"() -> ("Value"=w474:dbl[])  [unwired: 2 in, 2 out]
      n328 = property on="I2" class="Arr (strict)"() -> ("Value"=w477:dbl[])  [unwired: 2 in, 2 out]
      n329 = property on="ph2 45" class="Arr (strict)"() -> ("Value"=w476:dbl[])  [unwired: 2 in, 2 out]
      n330 = Build Cluster Array(w477, w476) -> (w478:cluster{dbl, dbl}[])
      n331 = Build Cluster Array(w475, w474) -> (w479:cluster{dbl, dbl}[])
      n332 = property on="Tab Control" class="TabCtl (strict)"("Value"=T2."Polar plot" ("Tab Control")) -> ()  [unwired: 2 in, 2 out]
      n333 = call <vilib>:"Polar Plot.vi"("data array [mag, phase (deg)]"=w479) -> ("new picture"=→"polar SLM1":picture)  [unwired: 10 in]
      n334 = call <vilib>:"Polar Plot.vi"("data array [mag, phase (deg)]"=w478) -> ("new picture"=→"polar SLM2":picture)  [unwired: 10 in]
    }
    frame #3 {
      n335 = property on="SupportFiles path" class="Path"() -> ("Value"=w496:path)  [unwired: 2 in, 2 out]
      n336 = script code="cd(Spath)\nComplexValuesLV"("A1_0"=w495, "A2_0"=w493, "Spath"=w496, "ph1"=w494, "ph2"=w492) -> ("C1"=w491:cdb[], "C2"=w487:cdb[])  [unwired: 1 in, 1 out]
      n337 = Complex To Polar(r * e^(i*theta)=w491) -> (r=w490:dbl[], theta=w489:dbl[])
      n338 = Complex To Polar(r * e^(i*theta)=w487) -> (r=w486:dbl[], theta=w485:dbl[])
      n339 = Build Cluster Array(w490, w489) -> (w488:cluster{dbl, dbl}[])
      n340 = Build Cluster Array(w486, w485) -> (w484:cluster{dbl, dbl}[])
      n341 = call <vilib>:"Polar Plot.vi"("data array [mag, phase (deg)]"=w484) -> ("new picture"=w482:picture)  [unwired: 10 in]
      n342 = call <vilib>:"Polar Plot.vi"("data array [mag, phase (deg)]"=w488) -> ("new picture"=w483:picture)  [unwired: 10 in]
      n343 = property on="polar SLM2" class="Pict"("Value"=w482) -> ()  [unwired: 2 in, 2 out]
      n344 = property on="polar SLM1" class="Pict"("Value"=w483) -> ()  [unwired: 2 in, 2 out]
    }
  }
